vi "Relative Sound Files.vi"() -> ()   [LabVIEW 2012]
panel:
  out "temperaturelimit":string="Sound\\XP Sounds\\tada.wav"
  out "xpexcl":string="Sound\\XP Sounds\\Windows XP Exclamation.wav"
  out "xpnotify":string="Sound\\XP Sounds\\Windows XP Notify.wav"
  out "xperror":string="Sound\\XP Sounds\\Windows XP Error.wav"
  out "xpding":string="Sound\\XP Sounds\\Windows XP Ding.wav"
  out "critstop":string="Sound\\XP Sounds\\Windows XP Critical Stop.wav"
  out "battlow":string="Sound\\XP Sounds\\Windows XP Battery Low.wav"
  out "battcrit":string="Sound\\XP Sounds\\Windows XP Battery Critical.wav"
  out "tada":string="Sound\\XP Sounds\\tada.wav"
  out "notify":string="Sound\\XP Sounds\\notify.wav"
  out "chord":string="Sound\\XP Sounds\\Chord.wav"
  out "ding":string="Sound\\XP Sounds\\ding.wav"
  out "startup":string="C:\\LabVIEW\\Sound\\Voice\\startup.wav"
  out "goodbye":string="Sound\\Voice\\goodbye.wav"
  out "train":string="Sound\\Voice\\train.wav"
  out "terminated":string="Sound\\Voice\\terminated.wav"
  out "notready":string="Sound\\Voice\\scan not ready.wav"
  out "scanint":string="Sound\\Voice\\scan interrupt.wav"
  out "scancancel":string="Sound\\Voice\\scan cancel.wav"
  out "error":string="Sound\\Voice\\error.wav"
  out "scanbelong":string="Sound\\Voice\\scan belong.wav"
  out "PClimit":string="Sound\\Voice\\PC limit.wav"
  out "pause":string="Sound\\Voice\\pause.wav"
  out "lowcryo":string="Sound\\Voice\\low cryogens.wav"
  out "danger":string="Sound\\Voice\\danger.wav"
  out "allscans":string="Sound\\Voice\\sweep interrupt.wav"
  out "scandone":string="Sound\\Voice\\scan done.wav"
  out "sweepint":string="Sound\\Voice\\sweep interrupt.wav"
  out "leavepersis":string="Sound\\Voice\\leave persistent.wav"
  out "enterpersis":string="Sound\\Voice\\enter persistent.wav"
  out "zero":string="Sound\\Voice\\at zero.wav"
  out "field":string="Sound\\Voice\\at field.wav"
  out "lvlN":string="Sound\\Voice\\N lvl hit.wav"
  out "lvlHe":string="Sound\\Voice\\He lvl hit.wav"
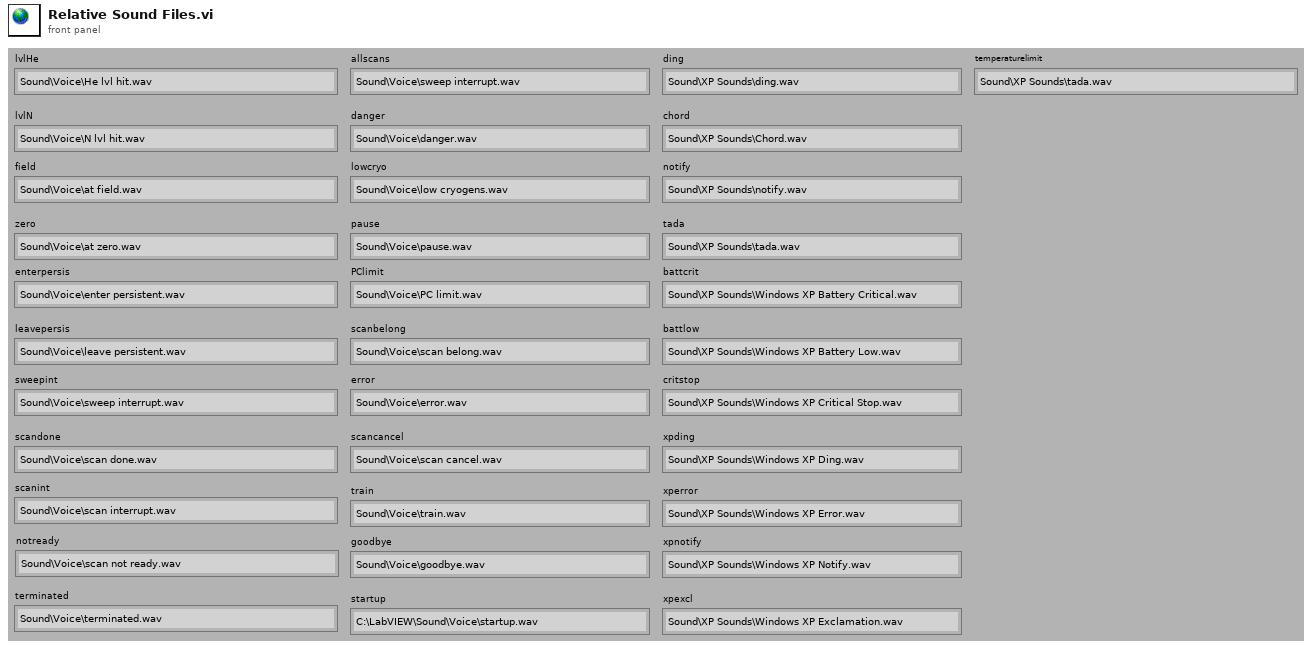
[diagram p1: front panel]
diagram:
